vi "Event Actor.vi"(10 "Spawn":refnum<class "Spawn.lvclass">, 11 "TEMPLATE Actor in":refnum<class "TEMPLATE Actor.lvclass">) -> (0 "Error out":errorcluster, 3 "TEMPLATE Actor out":refnum<class "TEMPLATE Actor.lvclass">)   [LabVIEW 2025, in "_Template.lvlib" / "Templates.lvlib" / "TEMPLATE Actor.lvlib" / "TEMPLATE Actor.lvclass"]
uses:
  TEMPLATE Actor.lvclass
  C:/git/jettl/src/jettl/jettl/Actor/Actor/Actor.lvclass
  jettl/jettl/Spawn/Spawn/Spawn.lvclass
  Control Refs.ctl
  TEMPLATE Actor.lvclass/TEMPLATE Actor.ctl
  C:/git/jettl/src/jettl Tools/_Template/Templates/TEMPLATE Actor/TEMPLATE Actor/TEMPLATE Actor.lvclass
  C:/git/jettl/src/jettl/jettl/Stopped Msg/Stopped/Stopped.lvclass
  jettl/jettl/jettl.lvlib
  jettl/jettl/Transport/Event/Event.lvlib
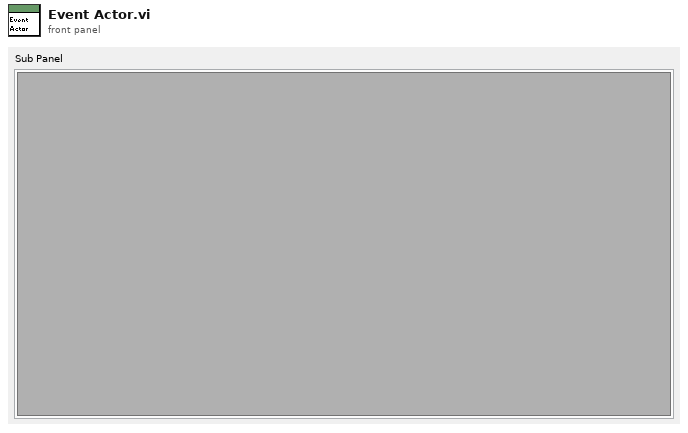
[diagram p1: front panel]
types:
  T1 = typedef "_Template.lvlib/Templates.lvlib/TEMPLATE Actor.lvlib/TEMPLATE Actor.lvclass/Control Refs.ctl" = cluster{"Sub Panel":refnum<vi>}
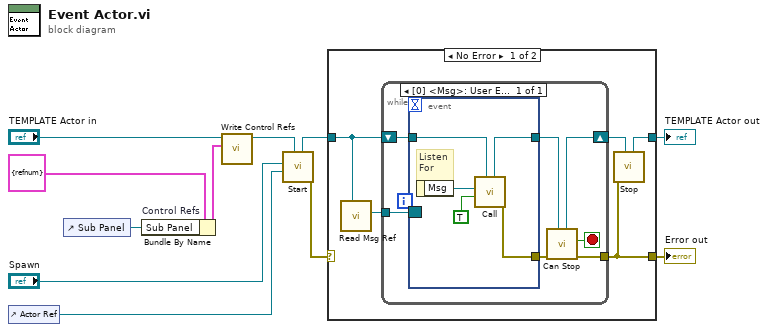
[diagram p0: block diagram]
diagram:
  n1 = control-ref of="Actor Ref"() -> (w6:refnum<vi>)
  n2 = control-ref of="Sub Panel"() -> (w1:refnum<vi>)
  n3 = Bundle By Name "Control Refs"(cluster=T1 {"Sub Panel"=refnum} ("Process Refs"), "Sub Panel"=w1) -> (w2:T1)
  n4 = call "Write Control Refs.vi"("Control Refs"=w2, "TEMPLATE Actor in"="TEMPLATE Actor in") -> ("TEMPLATE Actor out"=w3:refnum<class "TEMPLATE Actor.lvclass">)  [unwired: 9 in]
  n5 = call "Start.vi"("Actor in"=w3, "Actor Ref"=w6, "Spawn"="Spawn") -> ("Error out"=w8:errorcluster, "Actor out"=w7:refnum<class "TEMPLATE Actor.lvclass">)  [unwired: 7 in]
  n6 = case shown="No Error" w8 {
    selector: w8 -> [_ w29]
    tunnel: [w14 w30] -> w11
    tunnel: w7 -> [w13 w30]
    tunnel: [w16 w29] -> w10
    frame No Error {
      n7 = call "Read Msg Ref.vi"("Actor"=w13) -> ("Msg Ref"=w12:refnum<event-registration>)  [unwired: 10 in]
      n8 = while {
        shift-right: [w19] -> w15
        shift-left: w13 -> [w22]
        tunnel: w12 -> [w23]
        tunnel: [w20] -> w16
        stop <- w18 stop-if-true
        n9 = event shown="[0] <Msg>: User Event" {
          selector: w23 -> [_]
          dyn-events: _ -> [_]
          timeout: _ -> [_]
          tunnel: w22 -> [w28]
          tunnel: [w27] -> w17
          tunnel: [w25] -> w21
          event User Event {
            # "Listen\nFor"
            n10 = event-data() -> ("Msg"=w26:refnum<class "Msg.lvclass">)  [unwired: 1 in]
            n11 = call "Call.vi"("Actor in"=w28, "Listened To Msg"=TRUE, "Msg"=w26) -> ("Error out"=w25:errorcluster, "Actor out"=w27:refnum<class "TEMPLATE Actor.lvclass">)  [unwired: 6 in, 1 out]
          }
        }
        n12 = call "Can Stop.vi"("Actor in"=w17, "Error in"=w21) -> ("Error out"=w20:errorcluster, "Stop"=w18:bool, "Actor out"=w19:refnum<class "TEMPLATE Actor.lvclass">)  [unwired: 7 in]
      }
      n13 = call "Stop.vi"("Actor in"=w15, "Error in"=w16) -> ("Actor out"=w14:refnum<class "TEMPLATE Actor.lvclass">)  [unwired: 9 in]
    }
    frame Error {
    }
  }
  "TEMPLATE Actor out" <- w11
  "Error out" <- w10
